vi "sequence.vi"() -> ()   [LabVIEW 2019]
panel:
  out "temps pour deviner":dbl
  in  "nbre a trouver":dbl
  out "nbre testé":dbl
  out "nbre de i":dbl
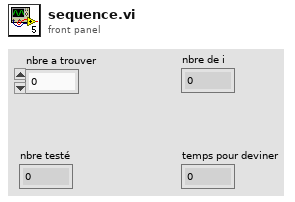
[diagram p1: front panel]
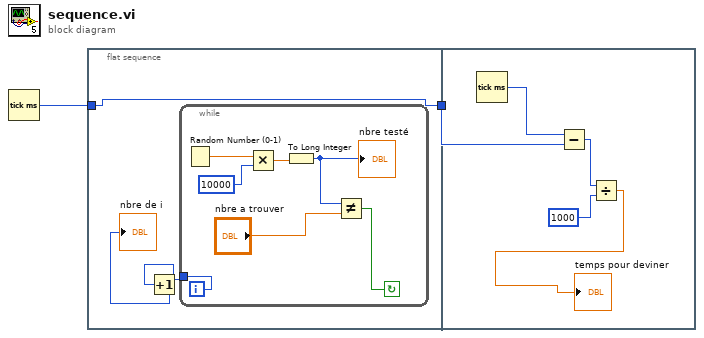
[diagram p0: block diagram]
diagram:
  n1 = Tick Count (ms)() -> (millisecond timer value=w2:u32)
  n2 = flat-sequence {
    tunnel: w2 -> [w5]
    tunnel: [w5] -> w1
    tunnel: w1 -> [w16]
    frame #0 {
      n3 = while {
        tunnel: [w8] -> w4
        i -> [w8]
        stop <- w9 continue-if-true
        n4 = Random Number (0-1)() -> (number: 0 to 1=w12:dbl)
        n5 = Multiply(x=w12, y=10000) -> (x*y=w10:dbl)
        n6 = To Long Integer(number=w10) -> (32bit integer=w7:i32)
        "nbre testé" <- w7
        n7 = Not Equal?(x=w7, y="nbre a trouver") -> (x != y?=w9:bool)
      }
      n8 = Increment(x=w4) -> (x+1=→"nbre de i":i32)
    }
    frame #1 {
      n9 = Tick Count (ms)() -> (millisecond timer value=w17:u32)
      n10 = Subtract(x=w17, y=w16) -> (x-y=w15:u32)
      n11 = Divide(x=w15, y=1000) -> (x/y=→"temps pour deviner":dbl)
    }
  }
